vi "MT_Test.vi"() -> ()   [LabVIEW 2020]
uses:
  <vilib>/Utility/inputDevices.llb/closeJoystick.vi
panel:
  out "键盘设备":refnum<k1>
  in  "退出":bool
  in  "Y绝对移动(mm)":dbl
  in  "X绝对移动(mm)":dbl
  in  "设置相对位置":bool
  in  "Y相对移动(μm)":dbl
  in  "X相对移动(μm)":dbl
  in  "设置绝对位置":bool
  out "当前Y轴位置(脉冲)":dbl
  out "当前X轴位置(脉冲)":dbl
  out "当前Y轴位置(mm)":dbl format="%.6f"
  out "当前X轴位置(mm)":dbl format="%#.6f"
  out "设备状态":bool
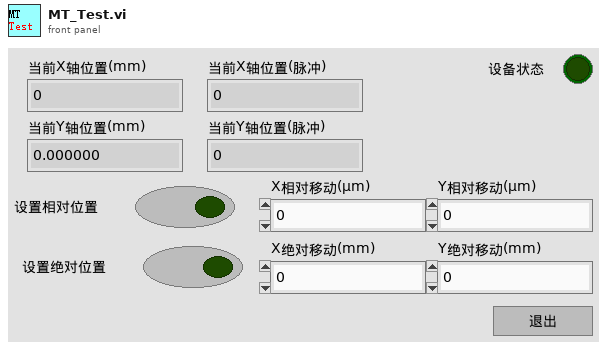
[diagram p1: front panel]
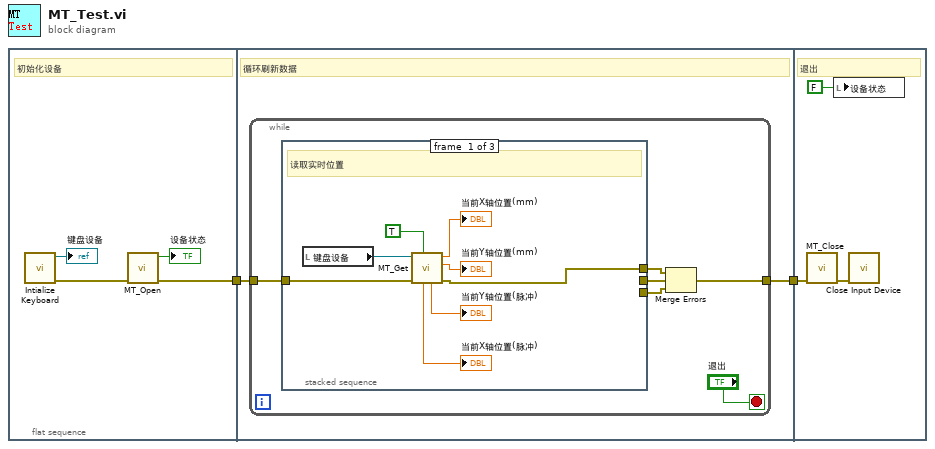
[diagram p0: block diagram]
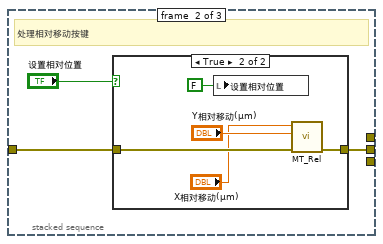
[diagram p2: hidden frame]
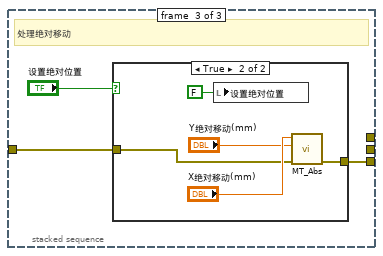
[diagram p4: hidden frame]
diagram:
  n1 = flat-sequence {
    tunnel: [w3] -> w2
    tunnel: w2 -> [w8]
    tunnel: [w7] -> w1
    tunnel: w1 -> [w42]
    frame #0 {
      # "初始化设备"
      n2 = call <vilib>:"Intialize Keyboard.vi"() -> ("error out"=w4:errorcluster, "device ID"=→"键盘设备":refnum<k1>)  [unwired: 10 in]
      n3 = call "MT_Open.vi"("Error In"=w4) -> ("Error Out"=w3:errorcluster, "MT设备状态"=→"设备状态":bool)  [unwired: 9 in]
    }
    frame #1 {
      # "循环刷新数据"
      n4 = while {
        tunnel: w8 -> [w13]
        tunnel: [w10] -> w7
        stop <- "退出" stop-if-true
        n5 = stacked-sequence {
          tunnel: w13 -> [w20 w24 w34]
          tunnel: [w17 _ _] -> w9
          tunnel: [_ w23 _] -> w12
          tunnel: [_ _ w32] -> w11
          frame #0 {
            # "读取实时位置"
            n6 = local read "键盘设备"() -> (w22:refnum<k1>)
            n7 = call "MT_Get.vi"("手动操作(False)"=TRUE, "Error In"=w20, "键盘设备输入"=w22) -> ("Error Out"=w17:errorcluster, "Y轴位置"=→"当前Y轴位置(mm)":dbl, "X轴位置"=→"当前X轴位置(mm)":dbl, "Y位置(脉冲)"=→"当前Y轴位置(脉冲)":dbl, "X位置(脉冲)"=→"当前X轴位置(脉冲)":dbl)  [unwired: 4 in]
          }
          frame #1 {
            # "处理相对移动按键"
            n8 = case shown="True" "设置相对位置" {
              tunnel: w24 -> [w26 w31]
              tunnel: [w26 w27] -> w23
              frame False {
              }
              frame True {
                n9 = local write "设置相对位置"(FALSE) -> ()
                n10 = call "MT_Rel.vi"("Error In"=w31, "Y轴偏移(μm)"="Y相对移动(μm)", "X轴偏移(μm)"="X相对移动(μm)") -> ("Error Out"=w27:errorcluster)  [unwired: 8 in]
              }
            }
          }
          frame #2 {
            # "处理绝对移动"
            n11 = case shown="True" "设置绝对位置" {
              tunnel: w34 -> [w35 w38]
              tunnel: [w35 w36] -> w32
              frame False {
              }
              frame True {
                n12 = local write "设置绝对位置"(FALSE) -> ()
                n13 = call "MT_Abs.vi"("X轴位置(mm)"="X绝对移动(mm)", "Y轴位置(mm)"="Y绝对移动(mm)", "Error In"=w38) -> ("Error Out"=w36:errorcluster)  [unwired: 7 in]
              }
            }
          }
        }
        n14 = Merge Errors(w9, w12, w11) -> (w10:errorcluster)
      }
    }
    frame #2 {
      # "退出"
      n15 = call "MT_Close.vi"("Error In"=w42) -> ("Error Out"=w41:errorcluster)  [unwired: 10 in]
      n16 = local write "设备状态"(FALSE) -> ()
      n17 = call-poly <vilib>:"Close Input Device.vi"("error in (no error)"=w41) -> ()  [unwired: 9 in, 1 out]
    }
  }
